vi "Log Test Program.vi"() -> ()   [LabVIEW 2018, in "Support Library.lvlib" / "Command Logging.lvlib"]
uses:
  Command Logging.lvlib
panel:
  out "error out":errorcluster
  in  "error in":errorcluster
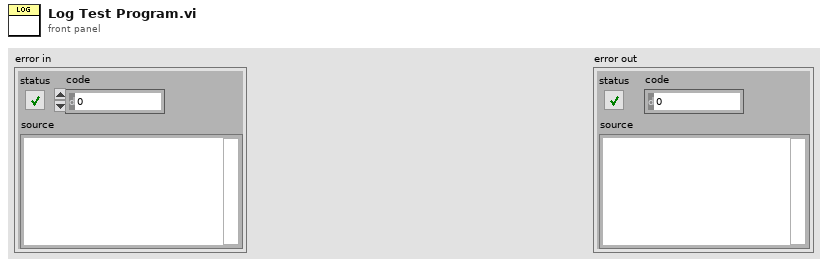
[diagram p1: front panel]
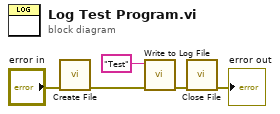
[diagram p0: block diagram]
diagram:
  n1 = call "Create File.vi"("error in"="error in") -> ("error out"=w5:errorcluster)  [unwired: 10 in]
  n2 = call "Write to Log File.vi"("error in"=w5, "text"="Test") -> ("error out"=w4:errorcluster)  [unwired: 9 in]
  n3 = call "Close File.vi"("error in"=w4) -> ("error out"=→"error out":errorcluster)  [unwired: 10 in]
